vi "Convert Lines To Polar.vi"(8 "Lines In":T1(array[cluster]) {"End Point"."Y" format="%.2f"; "End Point"."X" format="%.2f"; "Start Point"."Y" format="%.2f"; "Start Point"."X" format="%.2f"}, 10 "Angle In":dbl[](array[numeric]), 11 "Range In":dbl[](array[numeric])) -> (2 "Angle Out":dbl[](array[numeric]), 3 "Range Out":dbl[](array[numeric]))   [LabVIEW 2011]
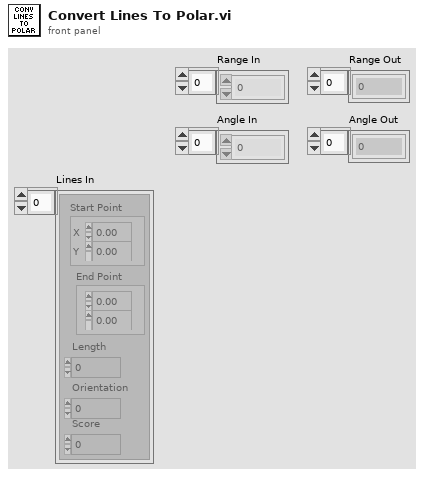
[diagram p1: front panel]
types:
  T1 = cluster{"Start Point":cluster{"X":sgl, "Y":sgl}, "End Point":cluster{"X":sgl, "Y":sgl}, "Length":dbl, "Orientation":dbl, "Score":dbl}[]
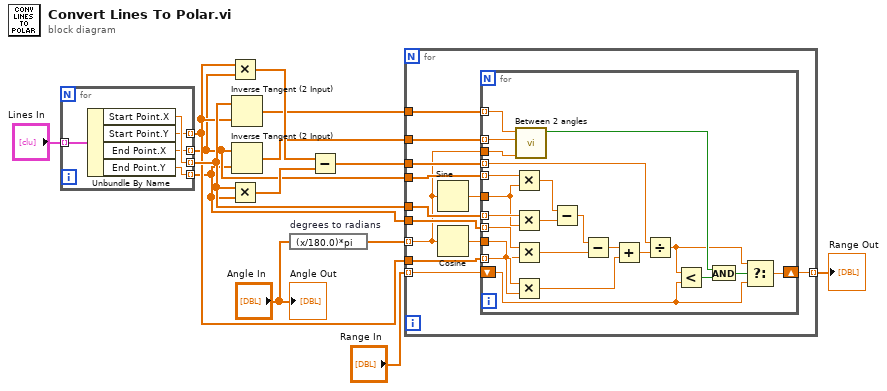
[diagram p0: block diagram]
diagram:
  n1 = for {
    tunnel: "Lines In" -> [w19] mode=indexing
    tunnel: [w18] -> w8 mode=indexing
    tunnel: [w17] -> w7 mode=indexing
    tunnel: [w16] -> w6 mode=indexing
    tunnel: [w15] -> w5 mode=indexing
    n2 = Unbundle By Name(w19) -> ("Start Point.X"=w18:sgl, "Start Point.Y"=w17:sgl, "End Point.X"=w16:sgl, "End Point.Y"=w15:sgl)
  }
  n3 = Multiply(x=w7, y=w6) -> (x*y=w13:sgl[])
  n4 = Multiply(x=w8, y=w5) -> (x*y=w14:sgl[])
  n5 = Inverse Tangent (2 Input)(1:w7, 2:w8) -> (0:w4:sgl[])
  n6 = Inverse Tangent (2 Input)(1:w5, 2:w6) -> (0:w3:sgl[])
  n7 = expression code="(x/180.0)*pi" "degrees to radians"("Angle In") -> (w10:dbl[])
  n8 = Subtract(x=w13, y=w14) -> (x-y=w11:sgl[])
  n9 = for {
    tunnel: w11 -> [w27]
    tunnel: w10 -> [w22] mode=indexing
    tunnel: "Range In" -> [w21] mode=indexing
    tunnel: w8 -> [w31]
    tunnel: w7 -> [w30]
    tunnel: w6 -> [w29]
    tunnel: w5 -> [w28]
    tunnel: w4 -> [w24]
    tunnel: w3 -> [w23]
    tunnel: [w20] -> w2 mode=indexing
    n10 = Sine(x=w22) -> (sin(x)=w25:dbl)
    n11 = Cosine(x=w22) -> (cos(x)=w26:dbl)
    n12 = for {
      tunnel: w31 -> [w54] mode=indexing
      tunnel: w30 -> [w53] mode=indexing
      tunnel: w29 -> [w50] mode=indexing
      tunnel: w28 -> [w51] mode=indexing
      tunnel: w27 -> [w42] mode=indexing
      tunnel: w26 -> [w52]
      tunnel: w25 -> [w49]
      tunnel: w24 -> [w40] mode=indexing
      tunnel: w23 -> [w39] mode=indexing
      tunnel: w22 -> [w38]
      shift-right: [w32] -> w20
      shift-left: w21 -> [w34]
      n13 = Multiply(x=w50, y=w49) -> (x*y=w48:dbl)
      n14 = Multiply(x=w54, y=w49) -> (x*y=w47:dbl)
      n15 = Multiply(x=w51, y=w52) -> (x*y=w45:dbl)
      n16 = Multiply(x=w53, y=w52) -> (x*y=w43:dbl)
      n17 = call "Between 2 angles.vi"("Test Angle"=w38, "Angle 2"=w39, "Angle 1"=w40) -> ("Is between Angle 1 and Angle 2"=w36:bool)  [unwired: 8 in]
      n18 = Subtract(x=w48, y=w47) -> (x-y=w46:dbl)
      n19 = Subtract(x=w46, y=w45) -> (x-y=w44:dbl)
      n20 = Add(x=w44, y=w43) -> (x+y=w41:dbl)
      n21 = Divide(x=w42, y=w41) -> (x/y=w33:dbl)
      n22 = Less?(x=w33, y=w34) -> (x < y?=w37:bool)
      n23 = And(x=w36, y=w37) -> (x .and. y?=w35:bool)
      n24 = Select(t=w33, s=w35, f=w34) -> (s? t:f=w32:dbl)
    }
  }
  "Range Out" <- w2
  "Angle Out" <- "Angle In"
